vi "Periodic Tasks.vi"(8 "error in":errorcluster) -> ()   [LabVIEW 2019]
doc: "This VI runs in parallel to other tasks. It can contain as many user-defined periodic loops as you need. These can carry out PID or other sorts of timed response."
uses:
  <vilib>/Rock Robotics/WPI/Utilities/WPI_GetSetVariantRefNum.vi
  <vilib>/Rock Robotics/Network Tables/NT Write Number.vi
  frc-software-2019/Transducer.ctl
panel:
  out "Transducer":i16
  out "PSI":dbl
  out "PSI Average":i32
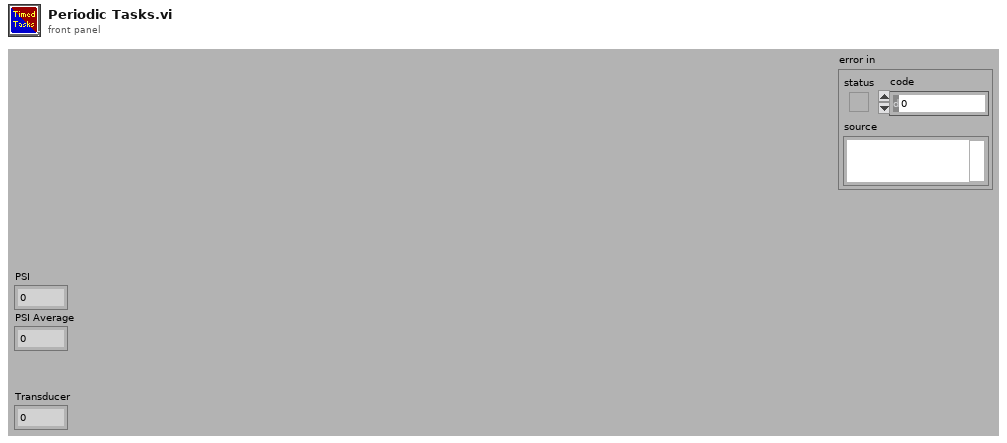
[diagram p1: front panel]
types:
  T1 = typedef "Transducer.ctl" = enum16{"Transducer"}
  T2 = typedef "WPI_AnalogChannelDevRef.ctl" = cluster{"DevStatus":errorcluster, "Analog Channel":T3}
  T3 = typedef "FPGA_AIChannel.ctl" = enum8{"AI 0", "AI 1", "AI 2", "AI 3", "AI MXP 0", "AI MXP 1", "AI MXP 2", "AI MXP 3", "Invalid"}
  T4 = typedef "WPI_JoystickDevRef.ctl" = cluster{"Device":T5}
  T5 = typedef "WPI_JoystickDeviceEnum.ctl" = enum16{"USB 0", "USB 1", "USB 2", "USB 3", "USB 4", "USB 5"}
  T6 = typedef "WPI_RobotDriveDevRef.ctl" = cluster{"DevStatus":errorcluster, "Motors[]":T7[], "Square Inputs":bool, "Max Output":dbl}
  T7 = typedef "WPI_MotorControlDeviceRef.ctl" = cluster{"DeviceStatus":errorcluster, "Type":T8, "PWM":cluster{"PWM Channel":T9, "DeadBand":T10}, "CAN":cluster{"Device Number":u8, "SetOutput VI Ref":variant, "GetOutput VI Ref":variant, "Enable VI Ref":variant, "Disable VI Ref":variant, "Data":variant}, "Invert":bool, "DIO PWM":cluster{"PWM \"Enable\" Channel":T9, "DIOChannel":T11, "PWM Rate":dbl}}
  T8 = typedef "WPI_MotorControlType.ctl" = enum16{"PWM", "CAN", "DIO PWM"}
  T9 = typedef "FPGA_DIOPWMChannel.ctl" = enum8{"PWM 0", "PWM 1", "PWM 2", "PWM 3", "PWM 4", "PWM 5", "PWM 6", "PWM 7", "PWM 8", "PWM 9", "PWM MXP 0", "PWM MXP 1", "PWM MXP 2", "PWM MXP 3", "PWM MXP 4", "PWM MXP 5", "PWM MXP 6", "PWM MXP 7", "PWM MXP 8", "PWM MXP 9", "Invalid"}
  T10 = typedef "WPI_PWMDeadband.ctl" = cluster{"Name":string, "maxPositivePwm":i32, "minPositivePwm":i32, "centerPwm":i32, "maxNegativePwm":i32, "minNegativePwm":i32, "angularRange":u16}
  T11 = typedef "FPGA_DIOChannel.ctl" = enum8{"DIO 0", "DIO 1", "DIO 2", "DIO 3", "DIO 4", "DIO 5", "DIO 6", "DIO 7", "DIO 8", "DIO 9", "DIO MXP 0", "DIO MXP 1", "DIO MXP 2", "DIO MXP 3", "DIO MXP 4", "DIO MXP 5", "DIO MXP 6", "DIO MXP 7", "DIO MXP 8", "DIO MXP 9", "DIO MXP 10", "DIO MXP 11", "DIO MXP 12", "DIO MXP 13", "DIO MXP 14", "DIO MXP 15", "SPI Port CS1", "SPI Port CS2", "SPI Port CS3", "SPI Port MISO", "SPI Port MOSI", "Invalid"}
  T12 = cluster{"JoystickDevRef":T4, "RobotDriveDevRef":T6}
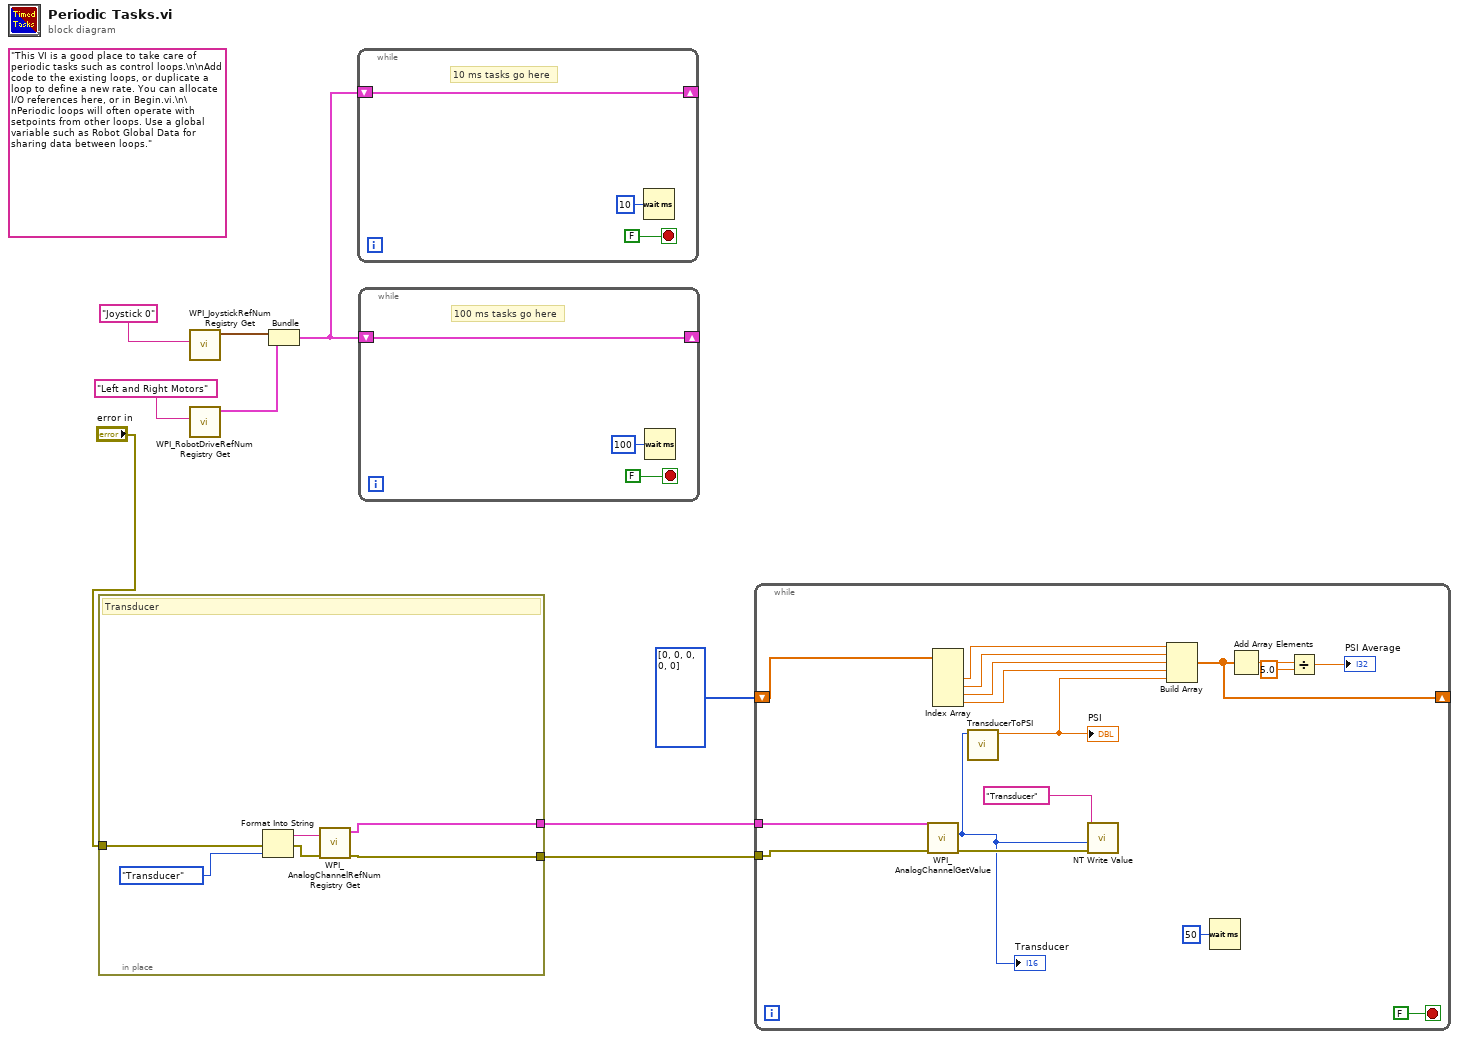
[diagram p0: block diagram]
diagram:
  (unwired) "This VI is a good place to take care of periodic tasks such as control loops.\n\nAdd code to the existing loops, or duplicate a loop to define a new rate. You can allocate I/O references here, or in Begin.vi.\n\nPeriodic loops will often operate with setpoints from other loops. Use a global variable such as Robot Global Data for sharing data between loops."
  n1 = in-place "In Place Element Structure" {
    in-place-border: "error in" -> [w13]
    in-place-border: [w11] -> w4
    in-place-border: [w10] -> w3
    # "Transducer"
    n2 = Format Into String(error in=w13, Transducer."Transducer" ("Enum")) -> (resulting string=w15:string, error out=w14:errorcluster)  [unwired: 2 in]
    n3 = call <vilib>:"WPI_AnalogChannelRefNum Registry Get.vi"("error in (no error)"=w14, "refnum name"=w15) -> ("error out"=w11:errorcluster, "AIDeviceRef"=w10:T2)  [unwired: 8 in]
  }
  n4 = call <vilib>:"WPI_JoystickRefNum Registry Get.vi"("refnum name"="Joystick 0") -> ("JoystickDevRef"=w7:T4)  [unwired: 1 in, 9 out]
  n5 = call <vilib>:"WPI_RobotDriveRefNum Registry Get.vi"("refnum name"="Left and Right Motors") -> ("RobotDriveDevRef"=w6:T6)  [unwired: 1 in, 9 out]
  n6 = Bundle("JoystickDevRef"=w7, "RobotDriveDevRef"=w6) -> (w5:T12)  [unwired: 1 out]
  n7 = while {
    shift-right: [w16] -> _
    shift-left: w5 -> [w16]
    stop <- FALSE stop-if-true
    # "10 ms tasks go here"
    n8 = Wait (ms)(milliseconds to wait=u32 10) -> ()  [unwired: 1 out]
  }
  n9 = while {
    shift-right: [w19] -> _
    shift-left: w5 -> [w19]
    stop <- FALSE stop-if-true
    # "100 ms tasks go here"
    n10 = Wait (ms)(milliseconds to wait=u32 100) -> ()  [unwired: 1 out]
  }
  n11 = while {
    tunnel: w4 -> [w38]
    tunnel: w3 -> [w37]
    shift-right: [w22] -> _
    shift-left: i32[] [0, 0, 0, 0, 0] -> [w31]
    stop <- FALSE stop-if-true
    n12 = call <vilib>:"WPI_AnalogChannelGetValue.vi"("error in (no error)"=w38, "AIDeviceRef"=w37) -> ("error out"=w36:errorcluster, "Value"=w32:i16)  [unwired: 7 in, 1 out]
    "Transducer" <- w32
    n13 = Index Array(array=w31) -> (element #2=w30:dbl, element #3=w29:dbl, element #4=w28:dbl, element #5=w27:dbl)  [unwired: 5 in, 1 out]
    n14 = call "TransducerToPSI.vi"("Transducer Input"=w32) -> ("PSI"=w26:dbl)  [unwired: 10 in]
    "PSI" <- w26
    n15 = call-poly <vilib>:"NT Write Value.vi"("error in"=w36, "Numeric"=w32, "Name"="Transducer") -> ()  [unwired: 8 in, 1 out]
    n16 = Build Array(w30, w29, w28, w27, w26) -> (w22:dbl[])
    n17 = Wait (ms)(milliseconds to wait=u32 50) -> ()  [unwired: 1 out]
    n18 = Add Array Elements(numeric array=w22) -> (sum=w25:dbl)
    n19 = Divide(x=w25, y=5.0) -> (x/y=→"PSI Average":dbl)
  }
